vi "ZLockSendRecv.vi"(8 "error in (no error)":errorcluster, 10 "parts":string[](array[string]), 11 "ZLock in":refnum<class "ZLock.lvclass">) -> (0 "error out":errorcluster, 2 "reply":string, 3 "ZLock out":refnum<class "ZLock.lvclass">)   [LabVIEW 2012, in "ZLock.lvclass"]
uses:
  <userlib>/BIAS2/subvis/zlock/ZLock.lvclass
  <userlib>/BIAS2/subvis/zlock/ZLock.lvclass/ZLock.ctl
  <vilib>/addons/zeromq/zeromq.lvlib
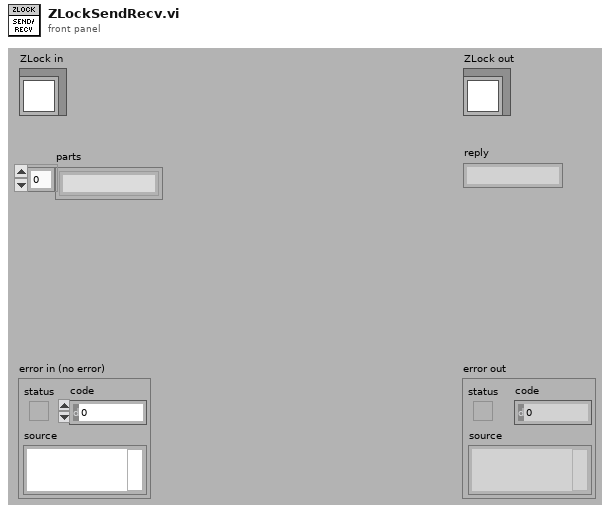
[diagram p1: front panel]
types:
  T1 = typedef "pointer.ctl" = u64
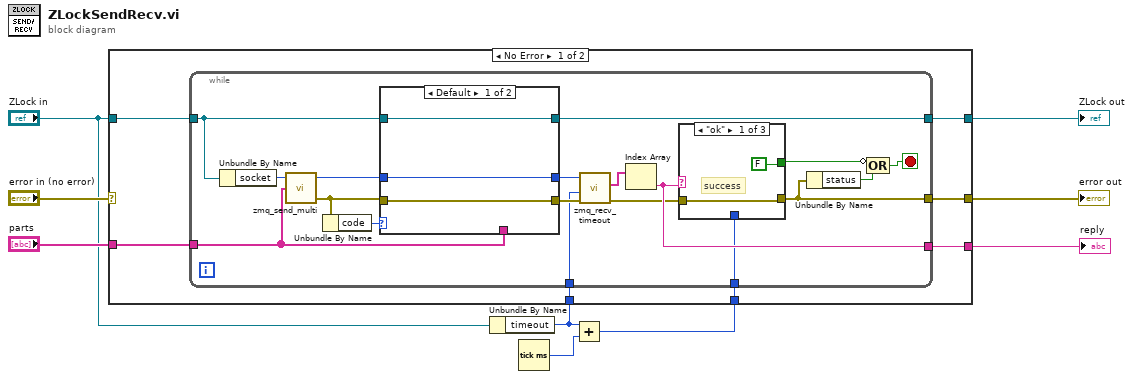
[diagram p0: block diagram]
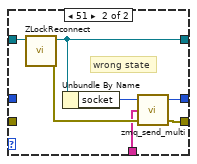
[diagram p2: hidden frame]
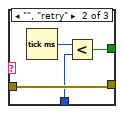
[diagram p3: hidden frame]
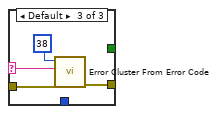
[diagram p4: hidden frame]
diagram:
  n1 = Unbundle By Name("ZLock in") -> ("timeout"=w1:i32)
  n2 = Tick Count (ms)() -> (millisecond timer value=w3:u32)
  n3 = Add(x=w1, y=w3) -> (x+y=w2:u32)
  n4 = case shown="No Error" "error in (no error)" {
    selector: "error in (no error)" -> [_ w56]
    tunnel: [w16 w56] -> w8
    tunnel: [w13 w55] -> w7
    tunnel: "ZLock in" -> [w14 w55]
    tunnel: "parts" -> [w12 _]
    tunnel: [w15 _] -> w5
    tunnel: w2 -> [w11 _]
    tunnel: w1 -> [w10 _]
    frame No Error {
      n5 = while {
        tunnel: [w22] -> w16
        tunnel: [w32] -> w15
        tunnel: w14 -> [w29]
        tunnel: [w27] -> w13
        tunnel: w12 -> [w26]
        tunnel: w11 -> [w18]
        tunnel: w10 -> [w17]
        stop <- w19 stop-if-true
        n6 = Unbundle By Name(w29) -> ("socket"=w34:T1)
        n7 = call <vilib>:"zmq_send_multi.vi"("parts"=w26, "socket in"=w34) -> ("error out"=w30:errorcluster, "socket out"=w25:T1)  [unwired: 2 in]
        n8 = Unbundle By Name(w30) -> ("code"=w31:i32)
        n9 = case shown="Default" w31 {
          tunnel: w30 -> [w37 _]
          tunnel: w29 -> [w36 w44]
          tunnel: [w37 w42] -> w28
          tunnel: [w36 w40] -> w27
          tunnel: w26 -> [_ w39]
          tunnel: w25 -> [w35 _]
          tunnel: [w35 w38] -> w24
          frame Default {
          }
          frame 51 {
            # "wrong state"
            n10 = call-dynamic "ZLockReconnect.vi"("ZLock in"=w44) -> ("error out"=w43:errorcluster, "ZLock out"=w40:refnum<class "ZLock.lvclass">)  [unwired: 9 in]
            n11 = Unbundle By Name(w40) -> ("socket"=w41:T1)
            n12 = call <vilib>:"zmq_send_multi.vi"("error in"=w43, "parts"=w39, "socket in"=w41) -> ("error out"=w42:errorcluster, "socket out"=w38:T1)  [unwired: 1 in]
          }
        }
        n13 = call <vilib>:"zmq_recv_timeout.vi"("error in"=w28, "timeout (ms)"=w17, "socket in"=w24) -> ("error out"=w23:errorcluster, "parts"=w33:string[])  [unwired: 1 in, 2 out]
        n14 = Index Array(array=w33) -> (element=w32:string)  [unwired: 1 in]
        n15 = case shown="\"ok\"" w32 {
          selector: w32 -> [_ _ w53]
          tunnel: w23 -> [w46 w50 w54]
          tunnel: [w46 w50 w51] -> w22
          tunnel: [FALSE w47 _] -> w21
          tunnel: w18 -> [_ w48 _]
          frame "ok" {
            # "success"
          }
          frame "", "retry" {
            n16 = Tick Count (ms)() -> (millisecond timer value=w49:u32)
            n17 = Less?(x=w49, y=w48) -> (x < y?=w47:bool)
          }
          frame Default {
            n18 = call <vilib>:"Error Cluster From Error Code.vi"("error in (no error)"=w54, "error message (\"\")"=w53, "error code (0)"=38) -> ("error out"=w51:errorcluster)  [unwired: 6 in]
          }
        }
        n19 = Unbundle By Name(w22) -> ("status"=w20:bool)
        n20 = Compound Arithmetic op=OR(invert w21, w20) -> (w19:bool)
      }
    }
    frame Error {
    }
  }
  "error out" <- w8
  "ZLock out" <- w7
  "reply" <- w5
